vi "Randomize_trials.vi"(0 "ArraySize":i32=100) -> (3 "Randomized":dbl[](array[numeric]))   [LabVIEW 2012]
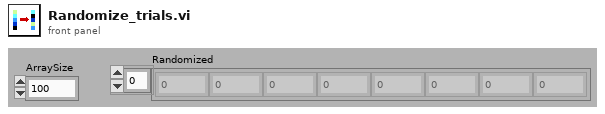
[diagram p1: front panel]
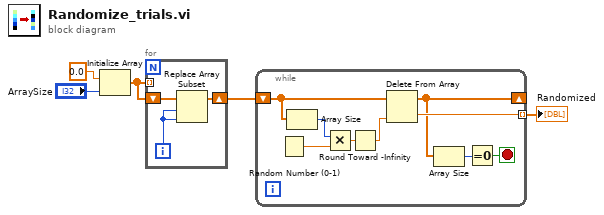
[diagram p0: block diagram]
diagram:
  n1 = Initialize Array(0.0 ("element"), "ArraySize") -> (w3:dbl[])
  n2 = for {
    tunnel: w3 -> [_] mode=indexing
    shift-right: [w7] -> w2
    shift-left: w3 -> [w8]
    i -> [w6]
    n3 = Replace Array Subset(array=w8, new element=w6, index=w6) -> (w7:dbl[])
  }
  n4 = while {
    shift-right: [w11] -> _
    shift-left: w2 -> [w16]
    tunnel: [w15] -> w1 mode=indexing
    stop <- w9 stop-if-true
    n5 = Random Number (0-1)() -> (number: 0 to 1=w17:dbl)
    n6 = Array Size(array=w16) -> (size(s)=w12:i32)
    n7 = Multiply(x=w12, y=w17) -> (x*y=w14:dbl)
    n8 = Round Toward -Infinity(1:w14) -> (0:w13:dbl)
    n9 = Delete From Array(array=w16, index=w13) -> (deleted portion=w15:dbl, array with subset deleted=w11:dbl[])  [unwired: 1 in]
    n10 = Array Size(array=w11) -> (size(s)=w10:i32)
    n11 = Equal To 0?(x=w10) -> (x = 0?=w9:bool)
  }
  "Randomized" <- w1
